vi "Read Discrete Inputs Response.vi"(8 "error in":errorcluster, 10 "modbus data unit in":refnum<class "Modbus Data Unit.lvclass">) -> (0 "error out":errorcluster, 2 "Data":bool[](array[boolean]))   [LabVIEW 2021, in "Master Function Definition.lvclass"]
doc: "Decodes the response for the read discrete inputs function."
uses:
  Master Function Definition.lvclass
  Modbus Data Unit/Modbus Data Unit.lvclass
  Modbus Data Unit/Modbus Data Unit.lvclass/Modbus Data Unit.ctl
  Modbus Data Unit/Deconstruct PDU.vi
  Master Function Definition.lvclass/Master Function Definition.ctl
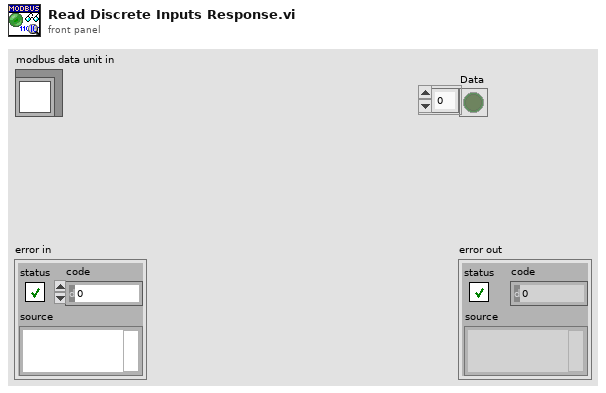
[diagram p1: front panel]
types:
  T1 = typedef "Modbus Data Unit.lvclass/Function.ctl" = u8
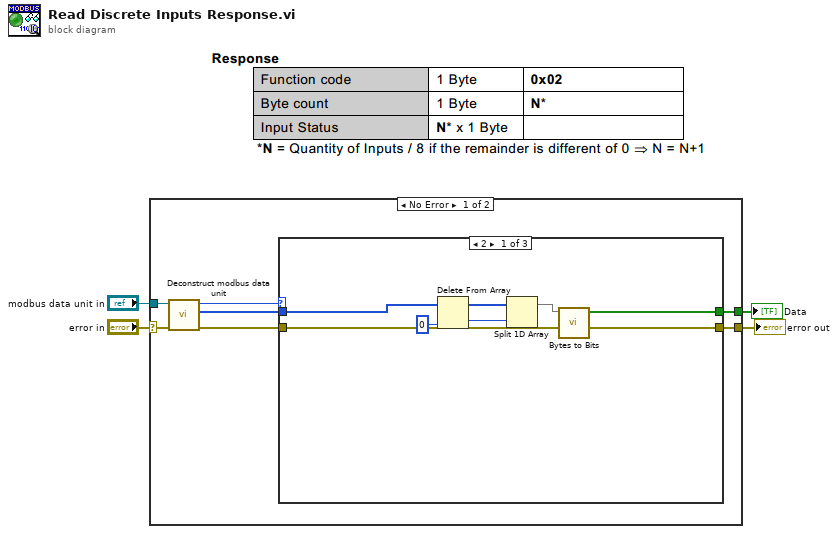
[diagram p0: block diagram]
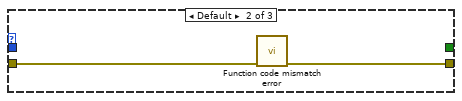
[diagram p2: hidden frame]
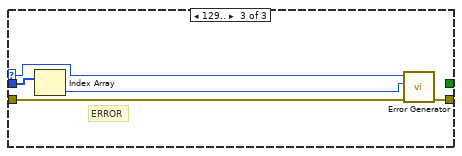
[diagram p3: hidden frame]
diagram:
  n1 = case shown="No Error" "error in" {
    selector: "error in" -> [w9 w26]
    tunnel: [w11 w26] -> w3
    tunnel: "modbus data unit in" -> [w7 _]
    tunnel: [w10 _] -> w1
    frame No Error {
      n2 = call "Deconstruct modbus data unit.vi"("error in"=w9, "modbus data unit in"=w7) -> ("error out"=w6:errorcluster, "data"=w8:u8[], "Function"=w5:T1)  [unwired: 7 in]
      n3 = case shown="2" w5 {
        selector: w5 -> [_ _ w21]
        tunnel: w6 -> [w16 w20 w22]
        tunnel: w8 -> [w18 _ w25]
        tunnel: [w16 w19 w24] -> w11
        tunnel: [w17 _ _] -> w10
        frame 2 {
          n4 = Delete From Array(array=w18, index=0) -> (deleted portion=w13:u8, array with subset deleted=w12:u8[])  [unwired: 1 in]
          n5 = Split 1D Array(array=w12, index=w13) -> (first subarray=w15:u8[])  [unwired: 1 out]
          n6 = call "Bytes to Bits.vi"("Bytes"=w15) -> ("Bits"=w17:bool[])  [unwired: 10 in]
        }
        frame Default {
          n7 = call "Function code mismatch error.vi"("error in (no error)"=w20) -> ("error out"=w19:errorcluster)  [unwired: 10 in]
        }
        frame 129.. {
          # "ERROR"
          n8 = Index Array(array=w25) -> (element=w23:u8)  [unwired: 1 in]
          n9 = call "Error Generator.vi"("error in"=w22, "data return (error code)"=w23, "function return"=w21) -> ("error out"=w24:errorcluster)  [unwired: 8 in]
        }
      }
    }
    frame Error {
    }
  }
  "error out" <- w3
  "Data" <- w1
